vi "Fix Velocities from Joysticks.vi"(10 "Axes":dbl[](array[numeric]), 11 "Deadband":cluster{"value":dbl, "value":dbl, "value":dbl}) -> (1 "Sending Input?":bool, 2 "Adjusted Robot Velocities":T1)   [LabVIEW 2020]
uses:
  swerve/Type Definitions/Data/Robot Velocities.ctl
  <vilib>/Rock Robotics/WPI/Joystick/XBox Axes Indexer.ctl
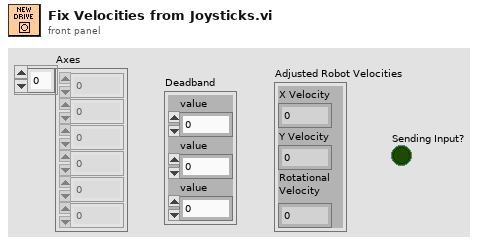
[diagram p1: front panel]
types:
  T1 = typedef "Robot Velocities.ctl" = cluster{"X Velocity":dbl, "Y Velocity":dbl, "Rotational \nVelocity":dbl}
  T2 = typedef "XBox Axes Indexer.ctl" = enum16{"Left X", "Left Y", "Left Trigger", "Right Trigger", "Right X", "Right Y"}
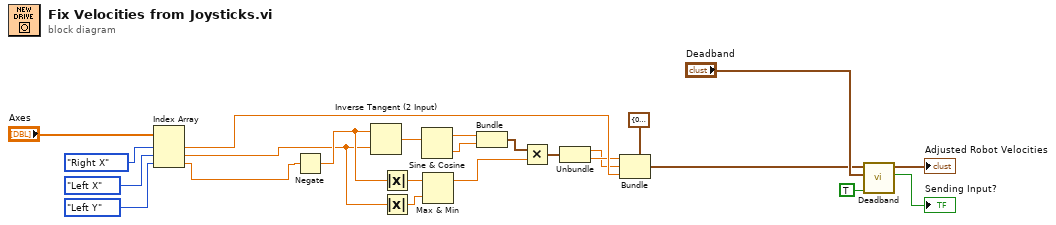
[diagram p0: block diagram]
diagram:
  n1 = Index Array(array="Axes", index #1=XBox_Axes_Indexer."Right X" ("XBox Axes"), index #2=XBox_Axes_Indexer."Left X" ("XBox Axes"), index #3=XBox_Axes_Indexer."Left Y" ("XBox Axes")) -> (element #1=w13:dbl, element #2=w2:dbl, element #3=w1:dbl)
  n2 = Negate(x=w1) -> (-x=w12:dbl)
  n3 = Inverse Tangent (2 Input)(1:w2, 2:w12) -> (0:w24:dbl)
  n4 = Absolute Value(x=w12) -> (abs(x)=w21:dbl)
  n5 = Absolute Value(x=w2) -> (abs(x)=w20:dbl)
  n6 = Sine & Cosine(0:w24) -> (1:w23:dbl, 2:w22:dbl)
  n7 = Max & Min(x=w21, y=w20) -> (max(x,y)=w18:dbl)  [unwired: 1 out]
  n8 = Bundle(w23, w22) -> (w19:cluster{dbl, dbl})  [unwired: 1 in]
  n9 = Multiply(x=w19, y=w18) -> (x*y=w14:cluster{dbl, dbl})
  n10 = Unbundle(w14) -> (w9:dbl, w10:dbl)
  n11 = Bundle(cluster=cluster{dbl, dbl, "upper limit":dbl} {0.0, 0.0, "upper limit"=0.0}, w10, w9, "upper limit"=w13) -> (w4:cluster{dbl, dbl, "upper limit":dbl})
  n12 = call "Deadband.vi"("Rescaling On?"=TRUE, "Deadband Info"="Deadband", "Robot Velocities"=w4) -> ("Sending Input?"=→"Sending Input?":bool, "Adjusted Robot Velocities"=→"Adjusted Robot Velocities":T1)  [unwired: 7 in]
